vi "Add Block Diagram Content.vi"(8 "error in (no error)":errorcluster, 9 "Term Refnums":refnum<vi>[](array[refnum]), 10 "ModuleLoop":T1, 11 "Quadrature Encoder Input in":refnum<class "Quadrature Encoder Input.lvclass">) -> (0 "error out":errorcluster, 3 "Quadrature Encoder Input out":refnum<class "Quadrature Encoder Input.lvclass">)   [LabVIEW 2025, in "Quadrature Encoder Input.lvclass"]
uses:
  Quadrature Encoder Input.lvclass
  VI/VI/Module.Refs.ctl
  <vilib>/Utility/miscctls.llb/LVPointTypeDef.ctl
  <vilib>/_script/New VI Object TypeDefs/NewVIObject_LVRelativePositionTypeDef.ctl
  <vilib>/_script/New VI Object TypeDefs/NewVIObject_LVRelativeDirectionTypeDef.ctl
  <vilib>/Utility/miscctls.llb/LVPoint32TypeDef.ctl
  Signal/Read IP Core Path.vi
  Signal/Read Signal Name.vi
  VI/VI/VI.lvclass
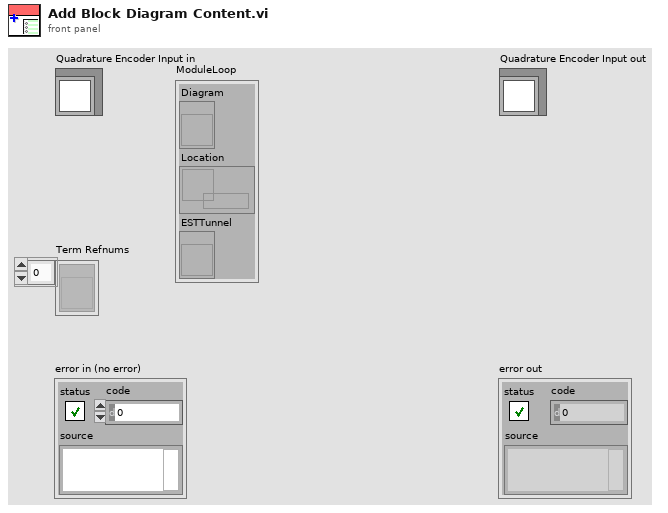
[diagram p1: front panel]
types:
  T1 = typedef "VI.lvclass/Module.Refs.ctl" = cluster{"Diagram":refnum<vi>, "Location":refnum<data-value>, "ESTTunnel":refnum<vi>}
  T2 = typedef "NewVIObject_LVRelativePositionTypeDef.ctl" = cluster{"Refnum":refnum<vi>, "Relative Direction":T3, "Point32":T4}
  T3 = typedef "NewVIObject_LVRelativeDirectionTypeDef.ctl" = enum32{"Right", "Left", "Top", "Bottom", "Top Right", "Top Left", "Bottom Right", "Bottom Left"}
  T4 = typedef "LVPoint32TypeDef.ctl" = cluster{"Horizontal":i32, "Vertical":i32}
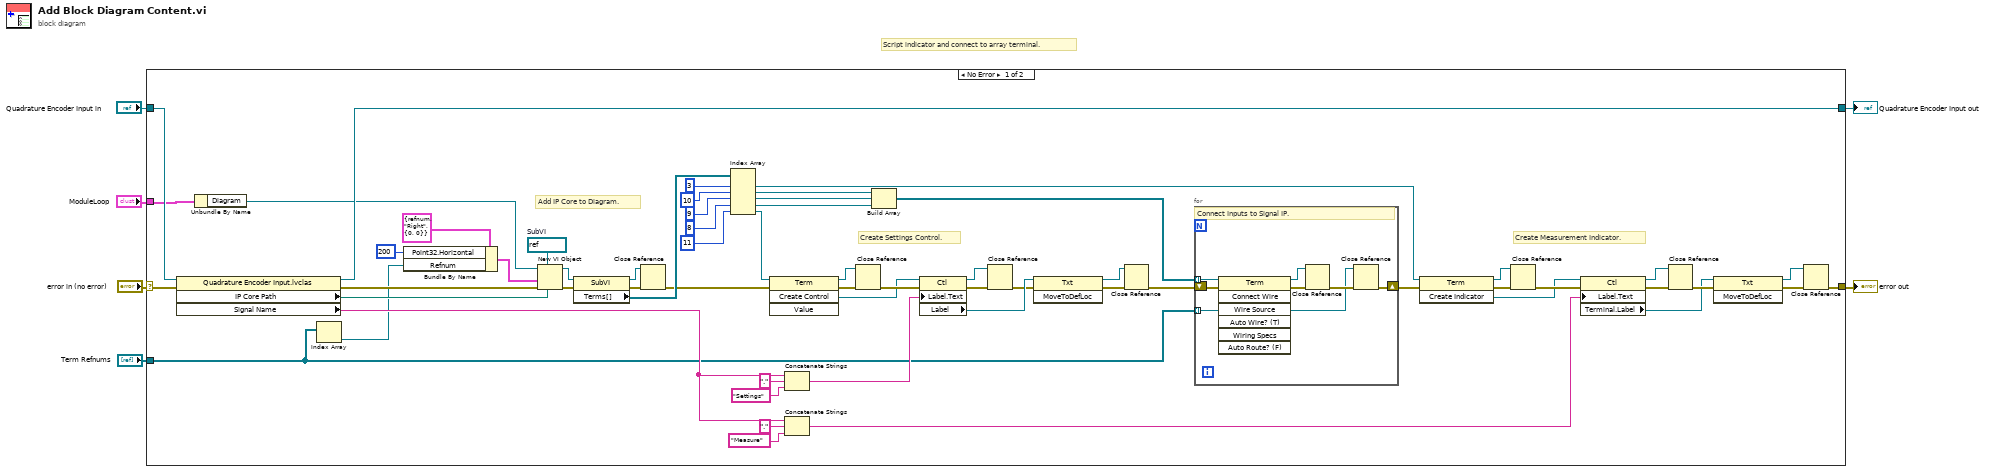
[diagram p0: block diagram]
diagram:
  # "Script indicator and connect to array terminal."
  n1 = case shown="No Error" "error in (no error)" {
    selector: "error in (no error)" -> [w19 w74]
    tunnel: "Quadrature Encoder Input in" -> [w66 w75]
    tunnel: [w65 w75] -> w1
    tunnel: "ModuleLoop" -> [w64 _]
    tunnel: [w23 w74] -> w2
    tunnel: "Term Refnums" -> [w14 _]
    frame No Error {
      w40 = refnum<vi> refnum  # SubVI
      # "Create Measurement Indicator."
      # "Create Settings Control."
      # "Add IP Core to Diagram."
      n2 = property class="Quadrature Encoder Input.lvclas"(reference=w66, error in=w19) -> (reference out=w65:refnum<class "Quadrature Encoder Input.lvclass">, error out=w24:errorcluster, "IP Core Path"=w21:path, "Signal Name"=w20:string)
      n3 = Unbundle By Name(w64) -> ("Diagram"=w22:refnum<vi>)
      n4 = Index Array(array=w14) -> (element=w15:refnum<vi>)  [unwired: 1 in]
      n5 = Bundle By Name(cluster=T2 {"Refnum"=refnum, "Relative Direction"=enum."Right", "Point32"={"Horizontal"=0, "Vertical"=0}} ("Relative Position"), "Point32.Horizontal"=200, "Refnum"=w15) -> (w25:T2)
      n6 = New VI Object(vi object class=w40, owner refnum=w22, position/next to=w25, 6:w21, 8:w24) -> (object refnum=w44:refnum<vi>, 0:w45:errorcluster)  [unwired: 3 in]
      n7 = property class="SubVI"(reference=w44, error in=w45) -> (reference out=w17:refnum<vi>, error out=w18:errorcluster, "Terms[]"=w41:refnum<vi>[])
      n8 = Close Reference(reference=w17, error in (no error)=w18) -> (error out=w16:errorcluster)
      n9 = Index Array(array=w41, index #1=3 ("index"), index #2=10 ("index"), index #3=9 ("index"), index #4=8 ("index"), index #5=11 ("index")) -> (element #1=w57:refnum<vi>, element #2=w49:refnum<vi>, element #3=w10:refnum<vi>, element #4=w9:refnum<vi>, element #5=w11:refnum<vi>)
      n10 = invoke class="Term" method="Create Control"(reference=w11, error in=w16) -> (reference out=w55:refnum<vi>, error out=w54:errorcluster, "Create Control"=w39:refnum<vi>)  [unwired: 2 in, 1 out]
      n11 = Concatenate Strings(w20, "." ("string"), "Settings" ("string")) -> (w46:string)
      n12 = Concatenate Strings(w20, "." ("string"), "Measure" ("string")) -> (w53:string)
      n13 = Close Reference(reference=w55, error in (no error)=w54) -> (error out=w56:errorcluster)
      n14 = Build Array(w49, w10, w9) -> (w13:refnum<vi>[])
      n15 = property class="Ctl"(reference=w39, error in=w56, "Label.Text"=w46) -> (reference out=w38:refnum<vi>, error out=w36:errorcluster, "Label"=w37:refnum<vi>)
      n16 = Close Reference(reference=w38, error in (no error)=w36) -> (error out=w35:errorcluster)
      n17 = invoke class="Txt" method="MoveToDefLoc"(reference=w37, error in=w35) -> (reference out=w33:refnum<vi>, error out=w34:errorcluster)  [unwired: 1 in, 1 out]
      n18 = Close Reference(reference=w33, error in (no error)=w34) -> (error out=w32:errorcluster)
      n19 = for {
        tunnel: w13 -> [w69] mode=indexing
        tunnel: w14 -> [w67] mode=indexing
        shift-right: [w73] -> w58
        shift-left: w32 -> [w68]
        # "Connect Inputs to Signal IP."
        n20 = invoke class="Term" method="Connect Wire"(reference=w69, error in=w68, "Wire Source"=w67) -> (reference out=w71:refnum<vi>, error out=w70:errorcluster)  [unwired: 4 in, 5 out]
        n21 = Close Reference(reference=w71, error in (no error)=w70) -> (error out=w72:errorcluster)
        n22 = Close Reference(reference=w67, error in (no error)=w72) -> (error out=w73:errorcluster)
      }
      n23 = invoke class="Term" method="Create Indicator"(reference=w57, error in=w58) -> (reference out=w61:refnum<vi>, error out=w62:errorcluster, "Create Indicator"=w50:refnum<vi>)  [unwired: 1 in]
      n24 = Close Reference(reference=w61, error in (no error)=w62) -> (error out=w63:errorcluster)
      n25 = property class="Ctl"(reference=w50, error in=w63, "Label.Text"=w53) -> (reference out=w59:refnum<vi>, error out=w60:errorcluster, "Terminal.Label"=w29:refnum<vi>)
      n26 = Close Reference(reference=w59, error in (no error)=w60) -> (error out=w30:errorcluster)
      n27 = invoke class="Txt" method="MoveToDefLoc"(reference=w29, error in=w30) -> (reference out=w28:refnum<vi>, error out=w31:errorcluster)  [unwired: 1 in, 1 out]
      n28 = Close Reference(reference=w28, error in (no error)=w31) -> (error out=w23:errorcluster)
    }
    frame Error {
    }
  }
  "error out" <- w2
  "Quadrature Encoder Input out" <- w1
